vi "Scripting_UpdateNewVI.vi"(0 "NewVI Ref or Path":variant, 1 "BaseClassNewVI Ref or Path(If empty the No base class will be used)":path, 5 "error in (no error)":errorcluster, 6 "AppRef":refnum<vi>) -> (19 "error out":errorcluster)   [LabVIEW 2020]
doc: "Update the NEW VI for GOOP4 templates"
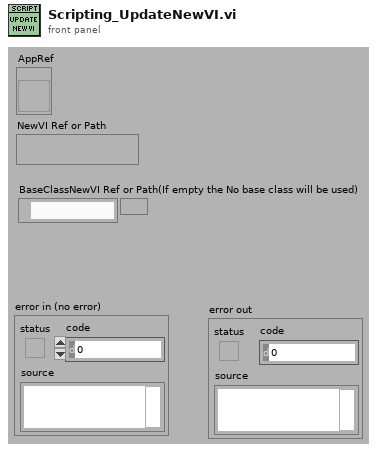
[diagram p1: front panel]
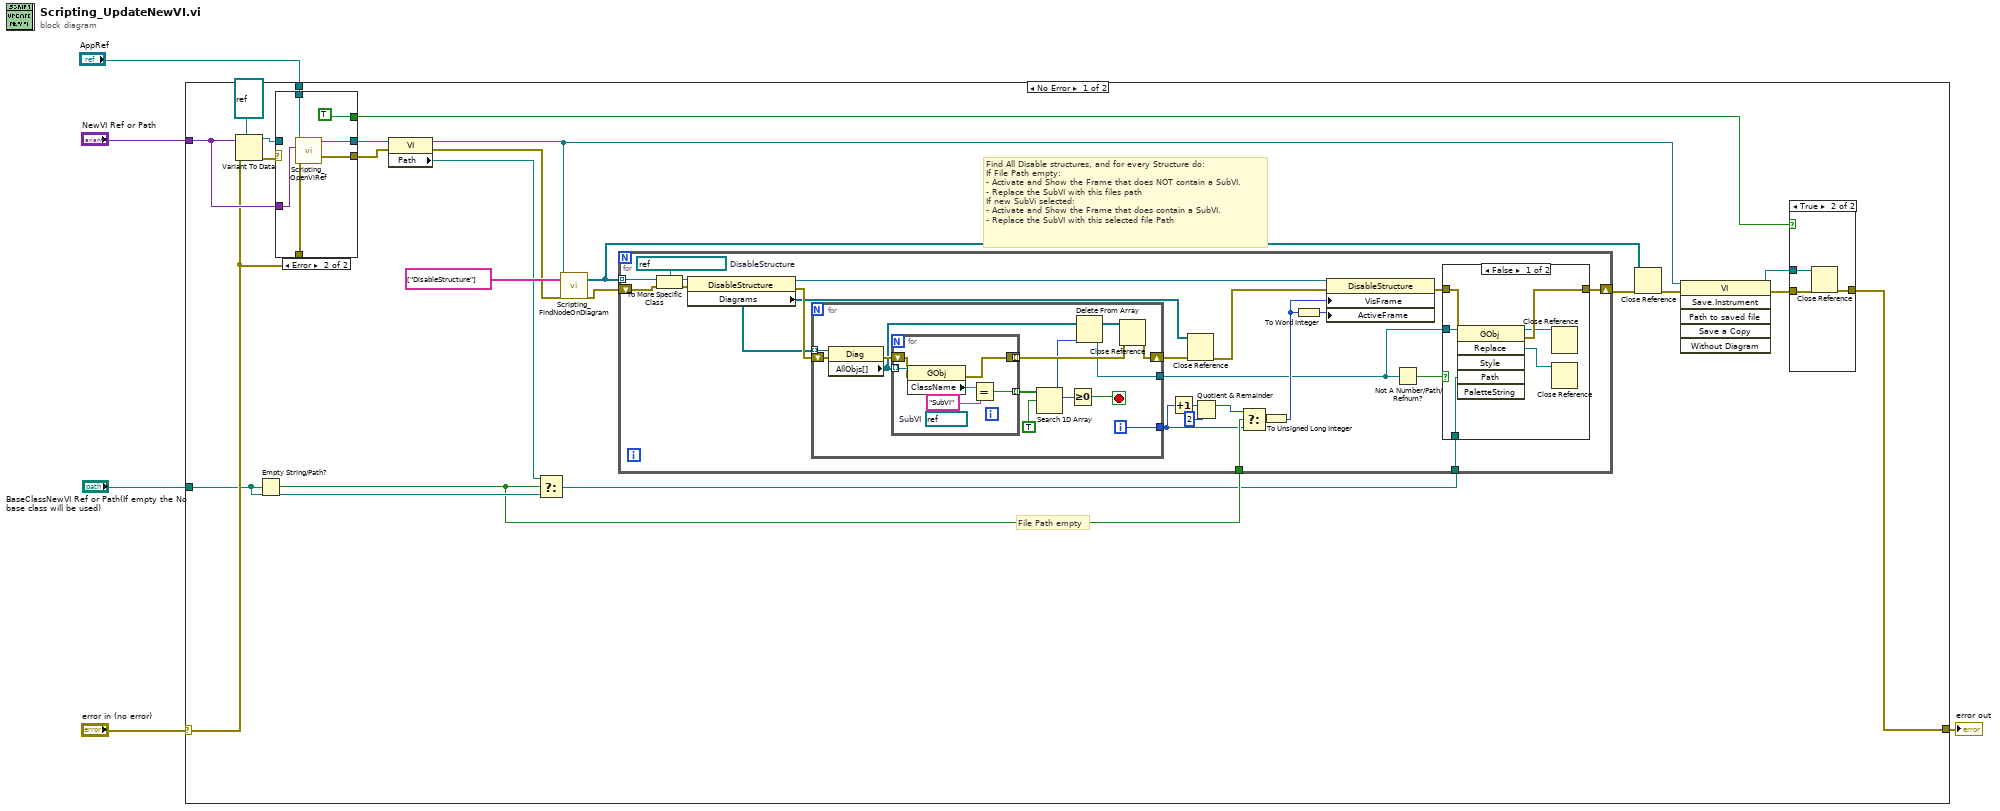
[diagram p0: block diagram]
diagram:
  n1 = case shown="No Error" "error in (no error)" {
    selector: "error in (no error)" -> [w19 w90]
    tunnel: [w28 w90] -> w5
    tunnel: "NewVI Ref or Path" -> [w23 _]
    tunnel: "BaseClassNewVI Ref or Path(If empty the No base class will be used)" -> [w17 _]
    tunnel: "AppRef" -> [w6 _]
    frame No Error {
      # "File Path empty"
      # "Find All Disable structures, and for every Structure do:\nIf File Path empty:\n- Activate and Show the Frame that does NOT contain a SubVI.\n- Replace the SubVI with this files path \nIf new SubVi selected:\n- Activate and Show the Frame that does contain a SubVI.\n- Replace the SubVI with this selected file Path"
      n2 = Variant To Data(error in=w19, type=refnum<vi> refnum ("ViRef(Ignored If Not Wired)"), Variant=w23) -> (data=w20:refnum<vi>, error out=w21:errorcluster)
      n3 = Empty String/Path?(string/path=w17) -> (empty?=w16:bool)
      n4 = case shown="Error" w21 {
        selector: w21 -> [w33 _]
        tunnel: w19 -> [_ w40]
        tunnel: w23 -> [_ w39]
        tunnel: w20 -> [w34 _]
        tunnel: [w34 w38] -> w9
        tunnel: [w33 w37] -> w7
        tunnel: [_ TRUE ("Front Panel Window:Open")] -> w10
        tunnel: w6 -> [_ w35]
        frame No Error {
        }
        frame Error {
          n5 = call <resource>:"Scripting_OpenViRef.vi"("error in"=w40, "ViPath/ViName/Viref"=w39, "AppRef"=w35) -> ("error out"=w37:errorcluster, "vi reference"=w38:refnum<vi>)  [unwired: 6 in, 1 out]
        }
      }
      n6 = property class="VI"(reference=w9, error in=w7) -> (reference out=w14:refnum<vi>, error out=w8:errorcluster, "Path"=w18:path)
      n7 = Select(t=w18, s=w16, f=w17) -> (s? t:f=w15:path)
      n8 = call <resource>:"Scripting_FindNodeOnDiagram.vi"("ViRef(Ignored If Not Wired)"=w14, "NodeTypesToSearchFor"=string[] ["DisableStructure"], "error in (no error)"=w8) -> ("Nodes"=w24:refnum<vi>[], "error out"=w26:errorcluster)  [unwired: 15 in]
      n9 = for {
        tunnel: w24 -> [w63] mode=indexing
        shift-right: [w44] -> w25
        shift-left: w26 -> [w61]
        tunnel: w16 -> [w56]
        tunnel: w15 -> [w46]
        w62 = refnum<vi> refnum  # DisableStructure
        n10 = To More Specific Class(target class=w62, reference=w63, error in=w61) -> (specific class reference=w60:refnum<vi>, error out=w59:errorcluster)
        n11 = property class="DisableStructure"(reference=w60, error in=w59) -> (reference out=w58:refnum<vi>, error out=w57:errorcluster, "Diagrams"=w41:refnum<vi>[])
        n12 = for {
          tunnel: w41 -> [w83] mode=indexing
          shift-right: [w75] -> w43
          shift-left: w57 -> [w81]
          tunnel: [w72] -> w47
          tunnel: [w71] -> w55
          i -> [w71]
          stop <- w73 stop-if-true
          n13 = property class="Diag"(reference=w83, error in=w81) -> (error out=w82:errorcluster, "AllObjs[]"=w78:refnum<vi>[])  [unwired: 1 out]
          n14 = for {
            tunnel: w78 -> [w89] mode=indexing
            tunnel: [w86] -> w80 mode=indexing
            shift-right: [w84] -> w76
            shift-left: w82 -> [w85]
            tunnel: [w84] -> _ mode=indexing
            (unwired) refnum<vi> refnum  # SubVI
            n15 = property class="GObj"(reference=w89, error in=w85) -> (error out=w84:errorcluster, "ClassName"=w88:string)  [unwired: 1 out]
            n16 = Equal?(x=w88, y="SubVI") -> (x = y?=w86:bool)
          }
          n17 = Search 1D Array(1D array=w80, element=TRUE) -> (index of element=w74:i32)  [unwired: 1 in]
          n18 = Greater Or Equal To 0?(x=w74) -> (x >= 0?=w73:bool)
          n19 = Delete From Array(array=w78, index=w74) -> (deleted portion=w72:refnum<vi>, array with subset deleted=w77:refnum<vi>[])  [unwired: 1 in]
          n20 = Close Reference(reference=w77, error in (no error)=w76) -> (error out=w75:errorcluster)
        }
        n21 = Increment(x=w55) -> (x+1=w54:i32)
        n22 = Close Reference(reference=w41, error in (no error)=w43) -> (error out=w42:errorcluster)
        n23 = Quotient & Remainder(x=w54, y=2) -> (x-y*floor(x/y)=w52:i32)  [unwired: 1 out]
        n24 = Select(t=w52, s=w56, f=w55) -> (s? t:f=w51:i32)
        n25 = To Unsigned Long Integer(number=w51) -> (unsigned 32bit integer=w50:u32)
        n26 = To Word Integer(number=w50) -> (16bit integer=w49:i16)
        n27 = property class="DisableStructure"(reference=w58, error in=w42, "VisFrame"=w50, "ActiveFrame"=w49) -> (error out=w45:errorcluster)  [unwired: 1 out]
        n28 = Not A Number/Path/Refnum?(number/path/refnum=w47) -> (NaN/Path/Refnum?=w48:bool)
        n29 = case shown="False" w48 {
          tunnel: w47 -> [w69 _]
          tunnel: w46 -> [w68 _]
          tunnel: w45 -> [w67 w70]
          tunnel: [w66 w70] -> w44
          frame False {
            n30 = invoke class="GObj" method="Replace"(reference=w69, error in=w67, "Path"=w68) -> (reference out=w65:refnum<vi>, error out=w66:errorcluster, "Replace"=w64:refnum<vi>)  [unwired: 3 in, 3 out]
            n31 = Close Reference(reference=w65) -> ()  [unwired: 1 in, 1 out]
            n32 = Close Reference(reference=w64) -> ()  [unwired: 1 in, 1 out]
          }
          frame True {
          }
        }
      }
      n33 = Close Reference(reference=w24, error in (no error)=w25) -> (error out=w13:errorcluster)
      n34 = invoke class="VI" method="Save.Instrument"(reference=w14, error in=w13) -> (reference out=w12:refnum<vi>, error out=w11:errorcluster)  [unwired: 4 in, 4 out]
      n35 = case shown="True" w10 {
        tunnel: [w29 w32] -> w28
        tunnel: w12 -> [_ w31]
        tunnel: w11 -> [w29 w30]
        frame False {
        }
        frame True {
          n36 = Close Reference(reference=w31, error in (no error)=w30) -> (error out=w32:errorcluster)
        }
      }
    }
    frame Error {
    }
  }
  "error out" <- w5
